vi "个性小灯一位数组循环移位.vi"() -> ()   [LabVIEW 2018]
panel:
  out "数组 2":T1[](array[typedef])
  in  "停止 2":bool
  in  "停止":bool
  out "数组":T2[](array[typedef])
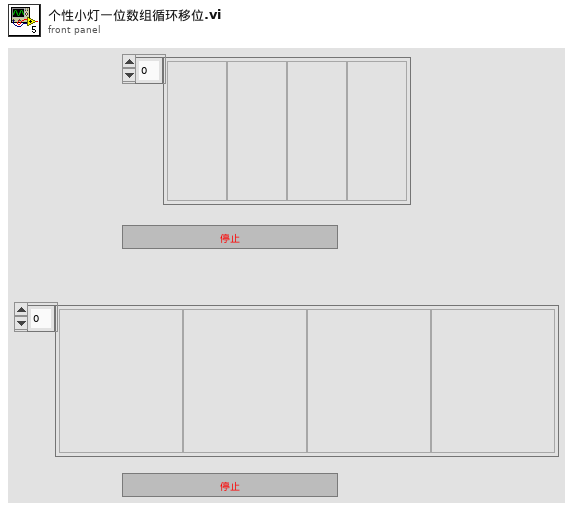
[diagram p1: front panel]
types:
  T1 = typedef "风扇.ctl" = bool
  T2 = typedef "小灯.ctl" = bool
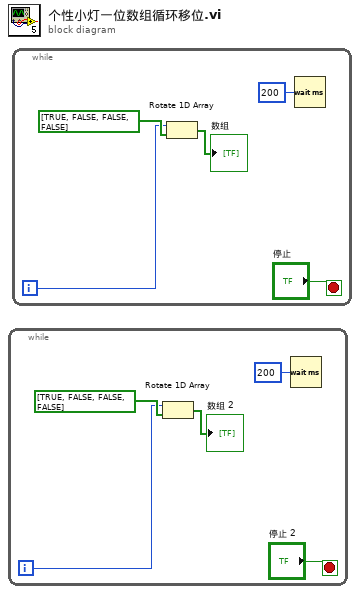
[diagram p0: block diagram]
diagram:
  n1 = while {
    i -> [w2]
    stop <- "停止 2" stop-if-true
    n2 = Rotate 1D Array(1:bool[] [TRUE, FALSE, FALSE, FALSE], 2:w2) -> (0:→"数组 2":bool[])
    n3 = Wait (ms)(milliseconds to wait=u32 200 ("等待时间（毫秒）")) -> ()  [unwired: 1 out]
  }
  n4 = while {
    i -> [w7]
    stop <- "停止" stop-if-true
    n5 = Rotate 1D Array(1:bool[] [TRUE, FALSE, FALSE, FALSE], 2:w7) -> (0:→"数组":bool[])
    n6 = Wait (ms)(milliseconds to wait=u32 200 ("等待时间（毫秒）")) -> ()  [unwired: 1 out]
  }
